vi "S2C_Access_ReadTypeCfg.vi"(8 "Error In":errorcluster) -> (0 "Error Out":errorcluster)   [LabVIEW 2015]
doc: "Reads the data contained within the Settings file and loads the data into VI specific global variables."
uses:
  Core/Command/S2C_CMD_Globals.vi
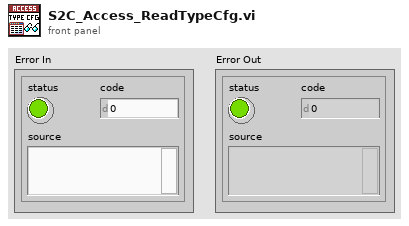
[diagram p1: front panel]
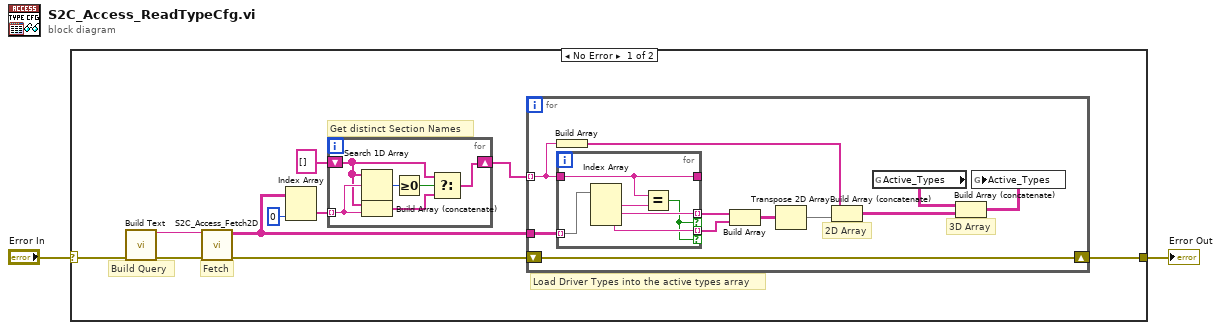
[diagram p0: block diagram]
diagram:
  n1 = case shown="No Error" "Error In" {
    selector: "Error In" -> [w3 w36]
    tunnel: [w4 w36] -> w1
    frame No Error {
      # "Load Driver Types into the active types array"
      # "Get distinct Section Names"
      # "Fetch"
      # "Build Query"
      n2 = call "Build Text"("error in (no error)"=w3) -> ("Result"=w10:string, "error out"=w12:errorcluster)  [unwired: 13 in]
      n3 = call "S2C_Access_Fetch2D.vi"("Error In"=w12, "Query"=w10) -> ("Error Out"=w11:errorcluster, "Data"=w9:string[][])  [unwired: 8 in]
      n4 = Index Array(array=w9, index (col)=0 ("disabled index (col)")) -> (element=w7:string[])  [unwired: 1 in]
      n5 = for {
        shift-right: [w13] -> w5
        shift-left: string[] [] -> [w15]
        tunnel: w7 -> [w16] mode=indexing
        n6 = Search 1D Array(1D array=w15, element=w16) -> (index of element=w18:i32)  [unwired: 1 in]
        n7 = Build Array (concatenate)(w15, w16) -> (w14:string[])
        n8 = Greater Or Equal To 0?(x=w18) -> (x >= 0?=w17:bool)
        n9 = Select(t=w15, s=w17, f=w14) -> (s? t:f=w13:string[])
      }
      n10 = for {
        tunnel: w9 -> [w29]
        shift-right: [w28] -> w4
        shift-left: w11 -> [w28]
        tunnel: w5 -> [w23] mode=indexing
        # "3D Array"
        # "2D Array"
        n11 = Build Array(w23) -> (w22:string[])
        n12 = for {
          tunnel: w29 -> [w35] mode=indexing
          tunnel: [w33] -> w25 mode=indexing if=w31
          tunnel: [w32] -> w24 mode=indexing if=w31
          tunnel: w23 -> [w30]
          tunnel: [w30] -> _
          n13 = Index Array(array=w35) -> (element #1=w34:string, element #2=w33:string, element #3=w32:string)  [unwired: 3 in]
          n14 = Equal?(x=w30, y=w34) -> (x = y?=w31:bool)
        }
        n15 = Build Array(w25, w24) -> (w26:string[][])
        n16 = Transpose 2D Array(2D array=w26) -> (transposed array=w27:string[][])
        n17 = Build Array (concatenate)(w22, w27) -> (w19:string[][])
        n18 = global read "S2C_CMD_Globals.vi" "Active_Types"() -> (w21:string[][][])
        n19 = Build Array (concatenate)(w21, w19) -> (w20:string[][][])
        n20 = global write "S2C_CMD_Globals.vi" "Active_Types"(w20) -> ()
      }
    }
    frame Error {
    }
  }
  "Error Out" <- w1
